vi "Configuration Tool Main.vi"() -> ()   [LabVIEW 2022 SP3, in "Configuration Tool.lvlib"]
doc: "This is the main VI for the configuration editor.Copyright 2017 National Instruments Corporation\n\nLicensed under the Apache License, Version 2.0 (the \"License\"); you may not use this file except in compliance with the License. You may obtain a copy of the License at http://www.apache.org/licenses/LICENSE-2.0\nUnless required by applicable law or agreed to in writing, software distributed under the License is distributed on an \"AS IS\" BASIS, WITHOUT WARRANTIES OR CONDITIONS OF ANY KIND, either express or implied. See the License for the specific language governing permissions and limitations under the License."
uses:
  Configuration Tool.lvlib
  Controls/StateCluster.ctl
  <vilib>/NI/Configuration Framework/Repository/NISE_CEF_Repository.lvclass
  <vilib>/NI/Configuration Framework/Node/NodeRef.ctl
  <vilib>/NI/Configuration Framework/Node/NISE_CEF_Node.lvclass
  <vilib>/NI/Configuration Framework/Node/StandardEvents.ctl
  <vilib>/NI/Configuration Framework/Node/UserEventRef.ctl
  <vilib>/NI/Configuration Framework/Controls/EventCluster.ctl
  <vilib>/NI/Configuration Framework/Node/NodeChangeEvent.ctl
  <vilib>/NI/Configuration Framework/Node/CacheState.ctl
  <vilib>/NI/Configuration Framework/Node/RefreshUIEvent.ctl
  <vilib>/NI/Configuration Framework/Node/StopEvent.ctl
  <vilib>/NI/Configuration Framework/glyph manager/glyph manager.ctl
  <vilib>/picture/picture.llb/imagedata.ctl
  Controls/AddMessage.ctl
  Controls/MoveMessage.ctl
  <vilib>/Utility/error.llb/DialogType.ctl
  Classes/cRIO Repo/BaseRepo.lvclass
  C:/Program Files (x86)/National Instruments/LabVIEW 2022/vi.lib/NI/Configuration Framework/Repository/NISE_CEF_Repository.lvclass
  Classes/BaseClass_class/BaseClass.lvclass
  <vilib>/Utility/sysdir.llb/System Directory Type.ctl
  <vilib>/NI/AMC/Create Single Message.vi
  <vilib>/NI/AMC/Update Message Routing Info.vi
  <vilib>/NI/AMC/Read Termination Message.vi
  <vilib>/NI/AMC/Send Message.vi
  <vilib>/NI/AMC/Globals.vi
  <vilib>/NI/AMC/AMC.lvlib
  <vilib>/NI/Configuration Framework/NISE_CEF_TreeControl.lvlib
  <vilib>/NI/Configuration Framework/glyph manager/glyph manager.lvlib
panel:
  in  "View":string(tree)
  in  "Exit":bool
  # "Configurator"
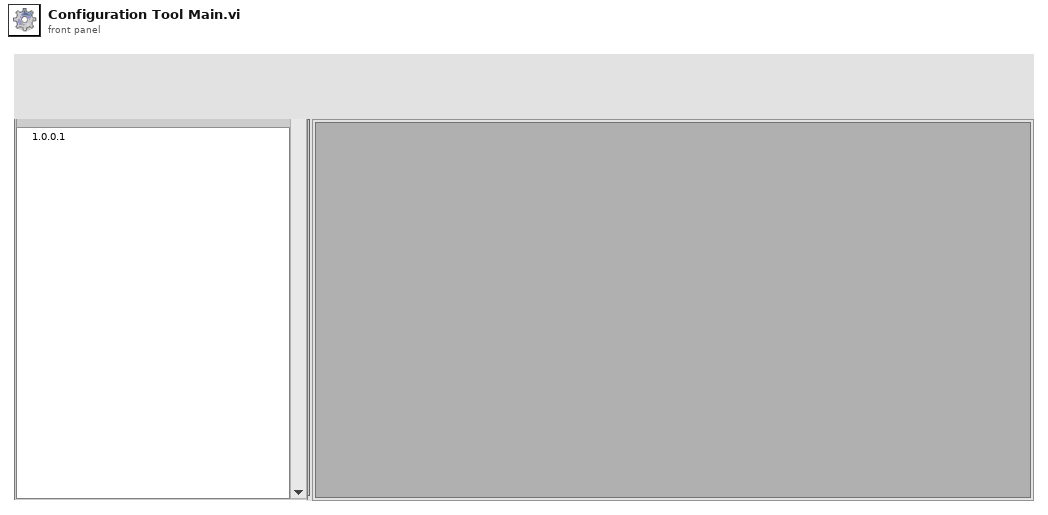
[diagram p1: front panel]
types:
  T1 = typedef "Configuration Tool.lvlib/StateCluster.ctl" = cluster{"repository":refnum<class "NISE_CEF_Repository.lvclass">, "root":T2, "unsaved changes":bool, "current path":path, "standard events":T3, "classes path":path, "glyph manager":T9}
  T2 = typedef "NISE_CEF_Node.lvclass/NodeRef.ctl" = refnum<data-value>
  T3 = typedef "NISE_CEF_Node.lvclass/StandardEvents.ctl" = cluster{"user event":T4, "node change":T5, "cache state":T6, "refresh UI":T7, "stop event":T8}
  T4 = typedef "NISE_CEF_Node.lvclass/UserEventRef.ctl" = refnum<user-event>
  T5 = typedef "NISE_CEF_Node.lvclass/NodeChangeEvent.ctl" = refnum<user-event>
  T6 = typedef "NISE_CEF_Node.lvclass/CacheState.ctl" = refnum<user-event>
  T7 = typedef "NISE_CEF_Node.lvclass/RefreshUIEvent.ctl" = refnum<user-event>
  T8 = typedef "NISE_CEF_Node.lvclass/StopEvent.ctl" = refnum<user-event>
  T9 = typedef "glyph manager.lvlib/glyph manager.ctl" = cluster{"search paths":path[], "glyph map":variant, "base glyphs":T10[], "desired overlays":string[]}
  T10 = typedef "imagedata.ctl" = cluster{"image type":i32, "image depth":i32, "image":u8[], "mask":u8[], "colors":u32[], "Rectangle":cluster{"left":i16, "top":i16, "right":i16, "bottom":i16}}
  T11 = typedef "AMC.lvlib/Message Queue.ctl" = refnum<queue>
  T12 = typedef "Configuration Tool.lvlib/AddMessage.ctl" = cluster{"node type":string, "to add to":string}
  T13 = typedef "Configuration Tool.lvlib/MoveMessage.ctl" = cluster{"node ref":T2, "new parent":T2, "Index":i32}
  T14 = typedef "Configuration Tool.lvlib/FilePaths.ctl" = cluster{"glyphs":path, "classes":path}
  T15 = typedef "DialogType.ctl" = u16
  T16 = typedef "System Directory Type.ctl" = i32
  T17 = typedef "NISE_CEF_Node.lvclass/Summary.ctl" = cluster{"ID":string, "parent ID":string, "node type":string, "text":string, "additional text":string, "glyph":string, "depth":i32, "glyph overlay":string}
  T18 = typedef "LVPoint32TypeDef.ctl" = cluster{"Horizontal":i32, "Vertical":i32}
  T19 = cluster{"data name":string, "drag data":variant}[]
  T20 = typedef "NISE_CEF_Node.lvclass/NodeMenuOptions.ctl" = cluster{"removable":bool, "movable":bool, "duplicate":bool}
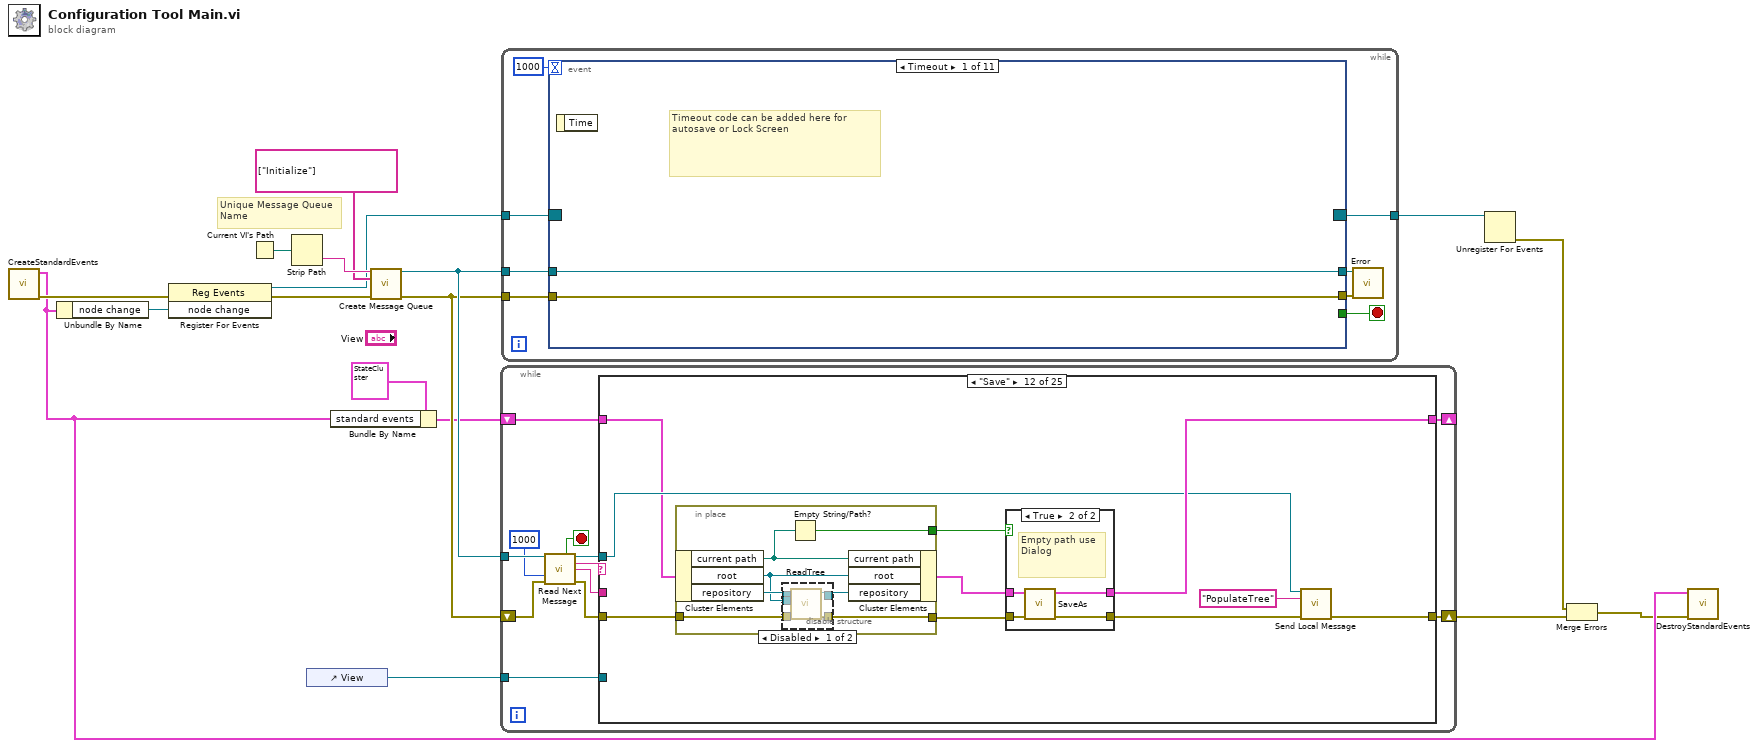
[diagram p0: block diagram]
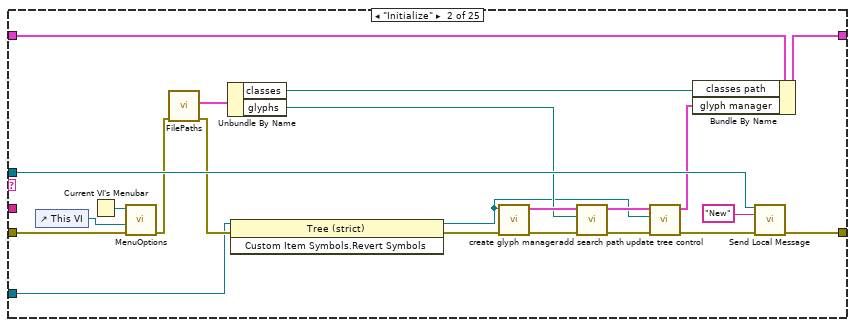
[diagram p3: hidden frame]
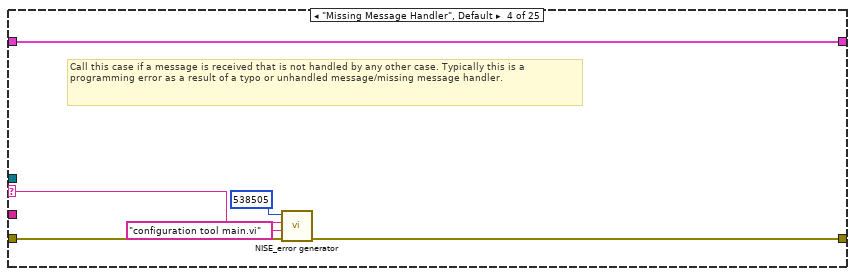
[diagram p5: hidden frame]
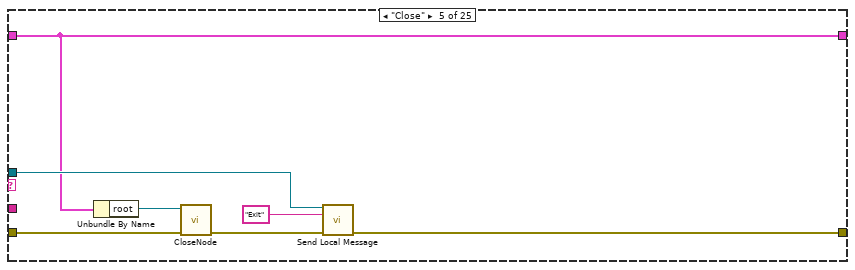
[diagram p6: hidden frame]
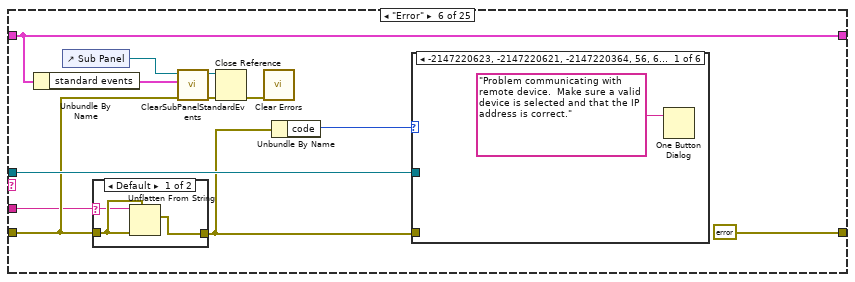
[diagram p7: hidden frame]
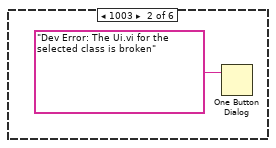
[diagram p9: hidden frame]
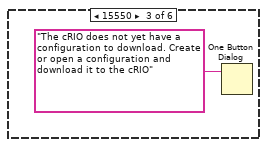
[diagram p10: hidden frame]
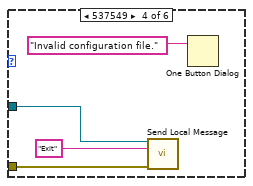
[diagram p11: hidden frame]
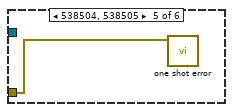
[diagram p12: hidden frame]
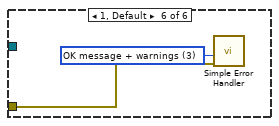
[diagram p13: hidden frame]
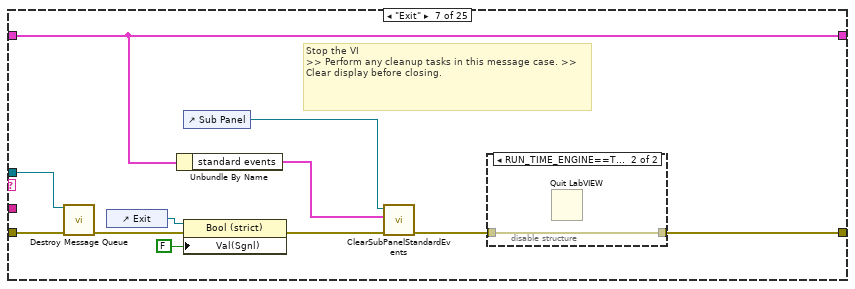
[diagram p14: hidden frame]
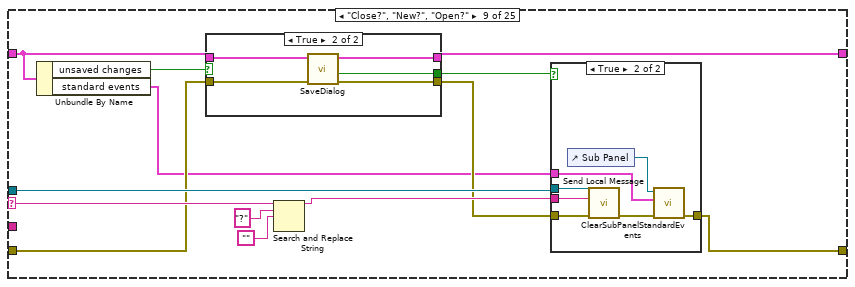
[diagram p17: hidden frame]
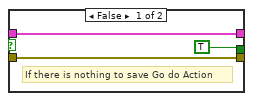
[diagram p18: hidden frame]
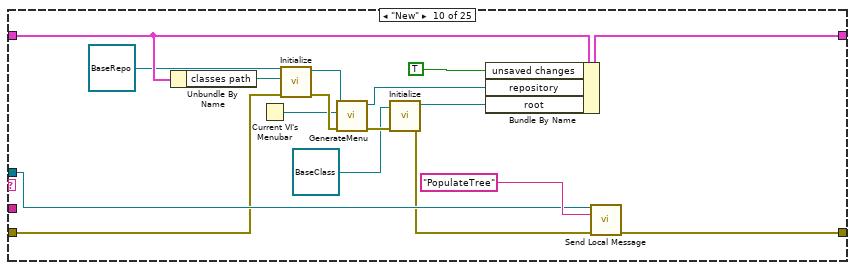
[diagram p20: hidden frame]
diagram:
  # "Unique Message Queue Name"
  n1 = call <vilib>:"CreateStandardEvents.vi"() -> ("error out"=w12:errorcluster, "standard events"=w6:T3)  [unwired: 10 in]
  n2 = Unbundle By Name(w6) -> ("node change"=w11:T5)
  n3 = register-events(error in=w12, w11) -> (reference out=w5:refnum<event-registration>, error out=w10:errorcluster)  [unwired: 1 in]
  n4 = Current VI's Path() -> (path=w16:path)
  n5 = Strip Path(path=w16) -> (name=w17:string)  [unwired: 1 out]
  n6 = control-ref of="View"() -> (w4:refnum<vi>)
  n7 = Bundle By Name(cluster=T1 {"repository"=refnum, "root"=refnum, "unsaved changes"=FALSE, "current path"=path "", "standard events"={"user event"=refnum, "node change"=refnum, "cache state"=refnum, "refresh UI"=refnum, "stop event"=refnum}, "classes path"=path "", "glyph manager"={"search paths"=[], "glyph map"=variant, "base glyphs"=[], "desired overlays"=[]}}, "standard events"=w6) -> (w8:T1)
  n8 = call <vilib>:"Create Message Queue.vi"("message queue name"=w17, "initial message names"=string[] ["Initialize"], "error in"=w10) -> ("message queue out"=w14:T11, "error out"=w13:errorcluster)  [unwired: 11 in]
  n9 = while "Message Processor" {
    shift-right: [w25] -> w7
    shift-left: w13 -> [w24]
    tunnel: w14 -> [w23]
    shift-right: [w21] -> _
    shift-left: w8 -> [w20]
    tunnel: w4 -> [w18]
    stop <- w29 stop-if-true
    n10 = call <vilib>:"Read Next Message.vi"("message queue in"=w23, "timeout (1 ms)"=1000, "error in"=w24) -> ("exit process?"=w29:bool, "message queue out"=w19:T11, "message name"=w28:string, "message value"=w27:string, "error out"=w26:errorcluster)  [unwired: 5 in, 3 out]
    n11 = case shown="\"Save\"" w28 {
      selector: w28 -> [_ _ _ w57 _ _ _ _ w118 _ _ _ _ _ _ _ _ w335 _ _ _ _ _ _ _]
      tunnel: w27 -> [_ _ _ _ _ w70 _ _ _ _ _ _ _ w246 _ w296 w313 w333 w385 w409 _ _ w449 w470 w477]
      tunnel: w26 -> [w31 w53 w55 w60 w63 w73 w105 w109 w111 w146 w162 w202 w233 w253 w273 w288 w312 w338 w387 w408 w430 w439 w448 w468 w478]
      tunnel: [w31 w49 w55 w58 w67 errorcluster {"status"=FALSE, "code"=0, "source"=""} ("error out") w97 w109 w122 w154 w158 w206 w235 w250 w273 w290 w316 w341 w389 w405 w424 w435 w445 w463 w476] -> w25
      tunnel: [w30 w45 w54 w61 w65 w77 w96 w108 w113 w152 w163 w209 w234 w247 w272 w282 w309 w342 w388 w410 w421 w438 w443 w471 w473] -> w21
      tunnel: w20 -> [w30 w46 w54 w61 w65 w77 w96 w108 w114 w149 w164 w204 w232 w248 w272 w286 w310 w342 w380 w410 w433 w438 w443 w471 w479]
      tunnel: w19 -> [_ w48 _ _ w66 w80 w104 _ w121 w153 w160 w205 _ w249 _ _ _ w336 _ _ _ _ w444 w462 w475]
      tunnel: w18 -> [_ w32 _ _ _ _ _ _ _ _ _ _ _ _ _ w283 w305 w330 w382 w403 w422 _ _ _ _]
      frame "------------Generic Operations------------" {
        # "Dummy case to add a seperation in the Case Structure menu"
      }
      frame "Initialize" {
        n12 = control-ref of="This VI"() -> (w52:refnum<vi>)
        n13 = Current VI's Menubar() -> (w51:refnum<k9>)
        n14 = call "MenuOptions.vi"("error in"=w53, "VI ref"=w52, "menu ref in"=w51) -> ("error out"=w44:errorcluster)  [unwired: 7 in, 1 out]
        n15 = call "FilePaths.vi"("error in"=w44) -> ("error out"=w35:errorcluster, "paths"=w47:T14)  [unwired: 9 in]
        n16 = Unbundle By Name(w47) -> ("classes"=w43:path, "glyphs"=w37:path)
        n17 = invoke class="Tree (strict)" method="Custom Item Symbols.Revert Symbols"(reference=w32, error in=w35) -> (reference out=w33:refnum<vi>, error out=w34:errorcluster)  [unwired: 1 in, 1 out]
        n18 = call <vilib>:"create glyph manager.vi"("error in"=w34, "tree ref (for default symbols)"=w33) -> ("error out"=w42:errorcluster, "glyph manager"=w41:T9)  [unwired: 8 in]
        n19 = call <vilib>:"add search path.vi"("error in"=w42, "search path"=w37, "glyph manager in"=w41) -> ("error out"=w40:errorcluster, "glyph manager out"=w39:T9)  [unwired: 7 in]
        n20 = call <vilib>:"update tree control.vi"("error in"=w40, "tree reference"=w33, "glyph manager in"=w39) -> ("error out"=w38:errorcluster, "glyph manager out"=w36:T9)  [unwired: 7 in]
        n21 = Bundle By Name(cluster=w46, "classes path"=w43, "glyph manager"=w36) -> (w45:T1)
        n22 = call <vilib>:"Send Local Message.vi"("message queue in"=w48, "message name"="New" ("Message Name"), "error in"=w38) -> ("error out"=w49:errorcluster)  [unwired: 10 in, 2 out]
      }
      frame "", "Idle" {
      }
      frame "Missing Message Handler", Default {
        # "Call this case if a message is received that is not handled by any other case. Typically this is a programming error as a result of a typo or unhandled message/missing message handler."
        n23 = call <vilib>:"NISE_error generator.vi"("error in"=w60, "source"="configuration tool main.vi", "append error message"=w57, "error code (0)"=538505) -> ("error out"=w58:errorcluster)  [unwired: 5 in]
      }
      frame "Close" {
        n24 = Unbundle By Name(w65) -> ("root"=w64:T2)
        n25 = call <vilib>:"CloseNode.vi"("error in"=w63, "node ref"=w64) -> ("error out"=w62:errorcluster)  [unwired: 9 in]
        n26 = call <vilib>:"Send Local Message.vi"("message queue in"=w66, "message name"="Exit", "error in"=w62) -> ("error out"=w67:errorcluster)  [unwired: 10 in, 2 out]
      }
      frame "Error" {
        n27 = Unbundle By Name(w77) -> ("standard events"=w69:T3)
        n28 = control-ref of="Sub Panel"() -> (w76:refnum<vi>)
        n29 = case shown="Default" w70 {
          selector: w70 -> [w82 _]
          tunnel: w73 -> [w83 w84]
          tunnel: [w81 w84] -> w72
          frame Default {
            n30 = Unflatten From String(type=w83, binary string=w82, error in (no error)=w83) -> (value=w81:errorcluster)  [unwired: 2 in, 2 out]
          }
          frame "" {
          }
        }
        n31 = call <vilib>:"ClearSubPanelStandardEvents.vi"("error in"=w73, "standard events"=w69, "sub panel ref in"=w76) -> ("error out"=w75:errorcluster, "sub panel ref out"=w74:refnum<vi>)  [unwired: 7 in]
        n32 = Close Reference(reference=w74, error in (no error)=w75) -> (error out=w71:errorcluster)
        n33 = call <vilib>:"Clear Errors.vi"("error in (no error)"=w71) -> ()  [unwired: 5 in, 2 out]
        n34 = Unbundle By Name(w72) -> ("code"=w78:i32)
        n35 = case shown="-2147220623, -2147220621, -2147220364, 56, 63" w78 {
          tunnel: w80 -> [_ _ _ w90 _ _]
          tunnel: w72 -> [_ _ _ w89 w92 w94]
          frame -2147220623, -2147220621, -2147220364, 56, 63 {
            n36 = One Button Dialog(message="Problem communicating with remote device.  Make sure a valid device is selected and that the IP address is correct.") -> ()  [unwired: 1 in, 1 out]
          }
          frame 1003 {
            n37 = One Button Dialog(message="Dev Error: The Ui.vi for the selected class is broken") -> ()  [unwired: 1 in, 1 out]
          }
          frame 15550 {
            n38 = One Button Dialog(message="The cRIO does not yet have a configuration to download. Create or open a configuration and download it to the cRIO") -> ()  [unwired: 1 in, 1 out]
          }
          frame 537549 {
            n39 = call <vilib>:"Send Local Message.vi"("message queue in"=w90, "message name"="Exit", "error in"=w89) -> ()  [unwired: 10 in, 3 out]
            n40 = One Button Dialog(message="Invalid configuration file.") -> ()  [unwired: 1 in, 1 out]
          }
          frame 538504, 538505 {
            n41 = call <vilib>:"one shot error.vi"("error in"=w92) -> ()  [unwired: 11 in]
          }
          frame 1, Default {
            w93 = T15 3 items=["no dialog", "OK message", "continue or stop message", "OK message + warnings", "continue/stop + warnings"] ("type of dialog (OK msg:1)")
            n42 = call <vilib>:"Simple Error Handler.vi"("type of dialog (OK msg:1)"=w93, "error in (no error)"=w94) -> ()  [unwired: 8 out]
          }
        }
      }
      frame "Exit" {
        # "Stop the VI                                                                             >> Perform any cleanup tasks in this message case. >> Clear display before closing."
        n43 = call <vilib>:"Destroy Message Queue.vi"("message queue in"=w104, "error in"=w105) -> ("error out"=w101:errorcluster)  [unwired: 11 in, 2 out]
        n44 = control-ref of="Exit"() -> (w103:refnum<vi>)
        n45 = Unbundle By Name(w96) -> ("standard events"=w95:T3)
        n46 = control-ref of="Sub Panel"() -> (w100:refnum<vi>)
        n47 = property class="Bool (strict)"(reference=w103, error in=w101, "Val(Sgnl)"=FALSE ("Exit")) -> (error out=w99:errorcluster)  [unwired: 1 out]
        n48 = call <vilib>:"ClearSubPanelStandardEvents.vi"("error in"=w99, "standard events"=w95, "sub panel ref in"=w100) -> ("error out"=w98:errorcluster)  [unwired: 7 in, 1 out]
        n49 = disable-structure shown="RUN_TIME_ENGINE==True" {
          disable-tunnel: [w106 w107] -> w97
          disable-tunnel: w98 -> [w106 w107]
          frame condition #0 (active) {
          }
          frame condition #1 {
            n50 = Quit LabVIEW() -> ()  [unwired: 1 in]
          }
        }
      }
      frame "------------Menu Operations--------------" {
        # "Dummy case to add a seperation in the Case Structure menu"
      }
      frame "Close?", "New?", "Open?" {
        n51 = Unbundle By Name(w114) -> ("unsaved changes"=w116:bool, "standard events"=w110:T3)
        n52 = case shown="True" w116 {
          tunnel: [TRUE ("SaveFlag") w130] -> w115
          tunnel: w114 -> [w124 w129]
          tunnel: [w124 w128] -> w113
          tunnel: w111 -> [w123 w127]
          tunnel: [w123 w126] -> w112
          frame False {
            # "If there is nothing to save Go do Action"
          }
          frame True {
            n53 = call "SaveDialog.vi"("error in"=w127, "state in"=w129) -> ("error out"=w126:errorcluster, "new"=w130:bool, "state out"=w128:T1)  [unwired: 7 in]
          }
        }
        n54 = Search and Replace String(input string=w118, search string="?", replace string="") -> (result string=w117:string)  [unwired: 5 in, 3 out]
        n55 = case shown="True" w115 {
          tunnel: w112 -> [w131 w138]
          tunnel: [w131 w134] -> w122
          tunnel: w121 -> [_ w137]
          tunnel: w117 -> [_ w136]
          tunnel: w110 -> [_ w132]
          frame False {
          }
          frame True {
            n56 = control-ref of="Sub Panel"() -> (w133:refnum<vi>)
            n57 = call <vilib>:"Send Local Message.vi"("message queue in"=w137, "message name"=w136, "error in"=w138) -> ("error out"=w135:errorcluster)  [unwired: 10 in, 2 out]
            n58 = call <vilib>:"ClearSubPanelStandardEvents.vi"("error in"=w135, "standard events"=w132, "sub panel ref in"=w133) -> ("error out"=w134:errorcluster)  [unwired: 7 in, 1 out]
          }
        }
      }
      frame "New" {
        n59 = Unbundle By Name(w149) -> ("classes path"=w148:path)
        n60 = Current VI's Menubar() -> (w141:refnum<k9>)
        n61 = call-dynamic "Initialize.vi"("error in"=w146, "path"=w148, "repository in"=refnum<class "BaseRepo.lvclass"> refnum ("BaseRepo.lvclass")) -> ("error out"=w145:errorcluster, "repository out"=w143:refnum<class "BaseRepo.lvclass">)  [unwired: 7 in]
        n62 = call-dynamic "GenerateMenu.vi"("error in"=w145, "menu ref in"=w141, "NISE_CEF_Repository in"=w143) -> ("error out"=w144:errorcluster, "NISE_CEF_Repository out"=w142:refnum<class "BaseRepo.lvclass">)  [unwired: 6 in, 1 out]
        n63 = call-dynamic "Initialize.vi"("error in"=w144, "cRIO in"=refnum<class "BaseClass.lvclass"> refnum ("BaseClass.lvclass")) -> ("error out"=w147:errorcluster, "data value reference"=w150:T2)  [unwired: 7 in, 1 out]
        n64 = Bundle By Name(cluster=w149, "unsaved changes"=TRUE ("SaveFlag"), "repository"=w142, "root"=w150) -> (w152:T1)
        n65 = call <vilib>:"Send Local Message.vi"("message queue in"=w153, "message name"="PopulateTree", "error in"=w147) -> ("error out"=w154:errorcluster)  [unwired: 10 in, 2 out]
      }
      frame "Open" {
        w157 = T16 0 items=["User Home"=0, "User Desktop"=1, "User Documents"=2, "User Application Data"=3, "User Preferences"=4, "User Temporary"=5, "Public Documents"=6, "Public Application Data"=7, "Public Preferences"=8, "Public Cache"=13, "System Core Libraries"=9, "System Installed Libraries"=10, "Application Files"=11, "Boot Volume Root"=12] ("system directory type")
        n66 = call <vilib>:"Get System Directory.vi"("system directory type"=w157) -> ("system directory"=w156:path)  [unwired: 10 in]
        n67 = in-place {
          in-place-border: w162 -> [w170]
          in-place-border: [w169] -> w159
          in-place-border: w156 -> [w165]
          n68 = in-place-cluster #1(w164) -> ("current path"=w167:path, "repository"=w178:refnum<class "NISE_CEF_Repository.lvclass">, "root"=w174:T2)  [unwired: 1 out]
          n69 = call "FileDialog.vi"("error in"=w170, "start path"=w165) -> ("error out"=w171:errorcluster, "cancelled"=w172:bool, "selected path"=w168:path)  [unwired: 7 in]
          n70 = Compound Arithmetic op=OR(invert w172) -> (w173:bool)
          n71 = case shown="True" w173 {
            tunnel: w178 -> [w179 w191]
            tunnel: [w179 w189] -> w176
            tunnel: [w180 w187] -> w169
            tunnel: [w181 w186] -> w175
            tunnel: w168 -> [_ w184]
            tunnel: w171 -> [w180 w183]
            tunnel: w174 -> [w181 w182]
            frame False {
            }
            frame True {
              n72 = call-dynamic "Open.vi"("error in"=w183, "file path"=w184, "repository in"=w191) -> ("error out"=w188:errorcluster, "invalid?"=w185:bool, "repository out"=w190:refnum<class "NISE_CEF_Repository.lvclass">)  [unwired: 6 in]
              n73 = case shown="False" w185 {
                tunnel: w190 -> [w196 w199]
                tunnel: [w195 w199] -> w189
                tunnel: w188 -> [w194 w198]
                tunnel: [w193 w198] -> w187
                tunnel: [w192 w197] -> w186
                tunnel: w182 -> [_ w197]
                frame False {
                  n74 = call-dynamic "WriteTree.vi"("error in"=w194, "repository in"=w196) -> ("error out"=w193:errorcluster, "root"=w192:T2, "repository out"=w195:refnum<class "NISE_CEF_Repository.lvclass">)  [unwired: 7 in]
                }
                frame True {
                }
              }
            }
          }
          n75 = Select(t=w167, s=w169, f=w168) -> (s? t:f=w166:path)
          n76 = in-place-cluster #1("current path"=w166, "unsaved changes"=FALSE ("SaveFlag"), "repository"=w176, "root"=w175) -> (w163:T1)
        }
        n77 = call <vilib>:"Send Local Message.vi"("message queue in"=w160, "message name"="PopulateTree", "error in"=w159) -> ("error out"=w158:errorcluster)  [unwired: 10 in, 2 out]
      }
      frame "Save" {
        n78 = in-place {
          in-place-border: w202 -> [w213]
          in-place-border: [w212] -> w201
          in-place-border: [w210] -> w200
          n79 = in-place-cluster #2(w204) -> ("current path"=w211:path, "root"=w214:T2, "repository"=w216:refnum<class "NISE_CEF_Repository.lvclass">)
          n80 = disable-structure shown="Disabled" {
            disable-tunnel: w216 -> [w221 _]
            disable-tunnel: [w220 _] -> w215
            disable-tunnel: w214 -> [w219 _]
            disable-tunnel: w213 -> [w218 _]
            disable-tunnel: [w217 _] -> w212
            frame Disabled {
              n81 = call-dynamic "ReadTree.vi"("error in"=w218, "root"=w219, "repository in"=w221) -> ("error out"=w217:errorcluster, "repository out"=w220:refnum<class "NISE_CEF_Repository.lvclass">)  [unwired: 7 in]
            }
            frame Enabled {
            }
          }
          n82 = Empty String/Path?(string/path=w211) -> (empty?=w210:bool)
          n83 = in-place-cluster #2("current path"=w211, "root"=w214, "repository"=w215) -> (w203:T1)
        }
        n84 = case shown="True" w200 {
          tunnel: w203 -> [w225 w227]
          tunnel: [w224 w226] -> w209
          tunnel: [w223 w228] -> w207
          tunnel: w201 -> [w222 w229]
          frame False {
            n85 = call "Save.vi"("error in"=w222, "state in"=w225) -> ("error out"=w223:errorcluster, "state out"=w224:T1)  [unwired: 8 in]
          }
          frame True {
            # "Empty path use Dialog"
            n86 = call "SaveAs.vi"("error in"=w229, "state in"=w227) -> ("error out"=w228:errorcluster, "state out"=w226:T1)  [unwired: 7 in, 1 out]
          }
        }
        n87 = call <vilib>:"Send Local Message.vi"("message queue in"=w205, "message name"="PopulateTree", "error in"=w207) -> ("error out"=w206:errorcluster)  [unwired: 10 in, 2 out]
      }
      frame "SaveAs" {
        n88 = in-place {
          in-place-border: w233 -> [w237]
          in-place-border: [w236] -> w231
          n89 = in-place-cluster #3(w232) -> ("root"=w238:T2, "repository"=w240:refnum<class "NISE_CEF_Repository.lvclass">)
          n90 = disable-structure shown="Disabled" {
            disable-tunnel: w240 -> [w245 _]
            disable-tunnel: [w244 _] -> w239
            disable-tunnel: w238 -> [w243 _]
            disable-tunnel: w237 -> [w242 _]
            disable-tunnel: [w241 _] -> w236
            frame Disabled {
              n91 = call-dynamic "ReadTree.vi"("error in"=w242, "root"=w243, "repository in"=w245) -> ("error out"=w241:errorcluster, "repository out"=w244:refnum<class "NISE_CEF_Repository.lvclass">)  [unwired: 7 in]
            }
            frame Enabled {
            }
          }
          n92 = in-place-cluster #3("root"=w238, "repository"=w239) -> (w230:T1)
        }
        n93 = call "SaveAs.vi"("error in"=w231, "state in"=w230) -> ("error out"=w235:errorcluster, "state out"=w234:T1)  [unwired: 7 in, 1 out]
      }
      frame "Custom View" {
        n94 = in-place {
          in-place-border: w253 -> [w260]
          in-place-border: [w259] -> w251
          in-place-border: w246 -> [w254]
          n95 = in-place-cluster #4(w248) -> ("repository"=w258:refnum<class "NISE_CEF_Repository.lvclass">, "root"=w257:T2)
          n96 = disable-structure shown="Disabled" {
            disable-tunnel: w260 -> [w271 _]
            disable-tunnel: [w270 _] -> w259
            disable-tunnel: w258 -> [w265 _]
            disable-tunnel: w257 -> [w264 _]
            disable-tunnel: [w263 _] -> w256
            disable-tunnel: [w262 _] -> w255
            disable-tunnel: w254 -> [w261 _]
            frame Disabled {
              n97 = call-dynamic "ReadTree.vi"("error in"=w271, "root"=w264, "repository in"=w265) -> ("error out"=w268:errorcluster, "repository out"=w267:refnum<class "NISE_CEF_Repository.lvclass">)  [unwired: 7 in]
              n98 = call-dynamic "CustomView.vi"("error in"=w268, "view name"=w261, "repository in"=w267) -> ("error out"=w269:errorcluster, "repository out"=w266:refnum<class "NISE_CEF_Repository.lvclass">)  [unwired: 7 in]
              n99 = call-dynamic "WriteTree.vi"("error in"=w269, "repository in"=w266) -> ("error out"=w270:errorcluster, "root"=w262:T2, "repository out"=w263:refnum<class "NISE_CEF_Repository.lvclass">)  [unwired: 7 in]
            }
            frame Enabled {
            }
          }
          n100 = in-place-cluster #4("repository"=w256, "root"=w255) -> (w247:T1)
        }
        n101 = call <vilib>:"Send Local Message.vi"("message queue in"=w249, "message name"="PopulateTree", "error in"=w251) -> ("error out"=w250:errorcluster)  [unwired: 10 in, 2 out]
      }
      frame "-------TreeControl Operations-----------" {
        # "Dummy case to add a seperation in the Case Structure menu"
      }
      frame "AddNode" {
        n102 = Unflatten From String(type=T12 {"node type"="", "to add to"=""} ("input cluster"), binary string=w296) -> (value=w294:T12)  [unwired: 3 in, 2 out]
        n103 = Unbundle By Name(w294) -> ("to add to"=w292:string, "node type"=w285:string)
        n104 = in-place {
          in-place-border: w288 -> [w302]
          in-place-border: [w301] -> w287
          in-place-border: w285 -> [w300]
          in-place-border: [w299] -> w284
          n105 = in-place-cluster #5(w286) -> ("repository"=w304:refnum<class "NISE_CEF_Repository.lvclass">)
          n106 = call-dynamic "GetClassPath.vi"("error in"=w302, "class name"=w300, "Repository in"=w304) -> ("error out"=w301:errorcluster, "class path"=w299:path, "Repository out"=w303:refnum<class "NISE_CEF_Repository.lvclass">)  [unwired: 6 in]
          n107 = in-place-cluster #5("repository"=w303) -> (w279:T1)
        }
        n108 = Unbundle By Name(w279) -> ("glyph manager"=w278:T9)
        n109 = call <vilib>:"Get LV Class Default Value.vi"("error in (no error)"=w287, "class path"=w284) -> ("error out"=w297:errorcluster, "object"=w298:refnum<class>)  [unwired: 8 in]
        n110 = To More Specific Class(target class=refnum<class "NISE_CEF_Node.lvclass"> refnum ("Node.lvclass"), reference=w298, error in=w297) -> (specific class reference=w280:refnum<class "NISE_CEF_Node.lvclass">, error out=w281:errorcluster)
        n111 = call-dynamic "AddGlyphtoGManager.vi"("error in"=w281, "glyph manager"=w278, "NISE_CEF_Node in"=w280) -> ("error out"=w276:errorcluster, "glyph manager out"=w277:T9, "NISE_CEF_Node out"=w275:refnum<class "NISE_CEF_Node.lvclass">)  [unwired: 6 in]
        n112 = call <vilib>:"AddNode.vi"("error in"=w276, "node in"=w275, "parent node ID"=w292) -> ("error out"=w291:errorcluster, "summary"=w289:T17[])  [unwired: 7 in]
        n113 = call <vilib>:"PopulateTreeSumaryWithGlyphManager.vi"("error in"=w291, "glyph manager"=w277, "summary"=w289, "tree ref in"=w283) -> ("error out"=w290:errorcluster, "glyph manager out"=w274:T9)  [unwired: 6 in]
        n114 = Bundle By Name(cluster=w279, "glyph manager"=w274) -> (w282:T1)
      }
      frame "Duplicate" {
        n115 = call <vilib>:"IDtoNode.vi"("error in"=w312, "ID"=w313) -> ("error out"=w314:errorcluster, "invalid Id"=w311:bool, "node ref"=w315:T2)  [unwired: 7 in]
        n116 = Unbundle By Name(w310) -> ("glyph manager"=w307:T9)
        n117 = case shown="False" w311 {
          tunnel: [w327 w329] -> w316
          tunnel: w315 -> [w326 _]
          tunnel: w314 -> [w323 w329]
          tunnel: w307 -> [w319 w328]
          tunnel: [w318 w328] -> w306
          tunnel: w305 -> [w317 _]
          frame False {
            n118 = call <vilib>:"DuplicateNode.vi"("same parent?"=TRUE ("s"), "error in"=w323, "node ref in"=w326) -> ("error out"=w324:errorcluster, "new node ref"=w325:T2)  [unwired: 7 in]
            n119 = call <vilib>:"Summary.vi"("error in"=w324, "node self ref"=w325) -> ("error out"=w321:errorcluster, "summary"=w320:T17[])  [unwired: 8 in]
            n120 = call <vilib>:"PopulateTreeSumaryWithGlyphManager.vi"("error in"=w321, "glyph manager"=w319, "summary"=w320, "tree ref in"=w317) -> ("error out"=w327:errorcluster, "glyph manager out"=w318:T9)  [unwired: 6 in]
          }
          frame True {
          }
        }
        n121 = Bundle By Name(cluster=w310, "unsaved changes"=TRUE, "glyph manager"=w306) -> (w309:T1)
      }
      frame "CustomMenuAction" {
        n122 = Match Pattern(string=w333, regular expression=":") -> (before substring=w332:string, after substring=w331:string)  [unwired: 1 in, 2 out]
        n123 = call <vilib>:"IDtoNode.vi"("error in"=w338, "ID"=w331) -> ("error out"=w339:errorcluster, "invalid Id"=w337:bool, "node ref"=w340:T2)  [unwired: 7 in]
        n124 = case shown="False" w337 {
          tunnel: [w348 w378] -> w341
          tunnel: w340 -> [w345 _]
          tunnel: w339 -> [w351 w378]
          tunnel: w336 -> [w352 _]
          tunnel: w335 -> [_ _]
          tunnel: w332 -> [w349 _]
          tunnel: w330 -> [w346 _]
          frame False {
            n125 = in-place {
              in-place-border: w352 -> [w376]
              in-place-border: w351 -> [w374]
              in-place-border: [w373] -> w347
              in-place-border: [w372] -> w350
              in-place-border: w349 -> [w371]
              in-place-border: w346 -> [w370]
              in-place-border: [w369] -> w344
              n126 = in-place-dvr #6(w345) -> (w377:refnum<class "NISE_CEF_Node.lvclass">)  [unwired: 1 out]
              n127 = call-dynamic "MenuHandler.vi"("tree control"=w370, "main message queue"=w376, "error in"=w374, "menu string"=w371, "NISE_CEF_Node in"=w377) -> ("error out"=w373:errorcluster, "refresh tree?"=w369:bool, "Unhandled"=w372:bool, "NISE_CEF_Node out"=w375:refnum<class "NISE_CEF_Node.lvclass">)  [unwired: 3 in]
              n128 = in-place-dvr #6(w375) -> (w343:T2)  [unwired: 1 out]
            }
            n129 = case shown="False" w350 {
              tunnel: w349 -> [_ w364]
              tunnel: [w356 w365] -> w348
              tunnel: w347 -> [w354 w366]
              tunnel: w344 -> [w353 _]
              tunnel: w343 -> [w355 _]
              frame False {
                n130 = case shown="True" w353 {
                  tunnel: [w357 w360] -> w356
                  tunnel: w355 -> [_ w359]
                  tunnel: w354 -> [w357 w358]
                  frame False {
                  }
                  frame True {
                    n131 = call <vilib>:"NodetoID.vi"("error in"=w358, "node ref"=w359) -> ("error out"=w362:errorcluster, "ID"=w363:string)  [unwired: 8 in]
                    n132 = call <vilib>:"Send Local Message.vi"("message name"="NodeDataChange", "message value"=w363, "error in"=w362) -> ("error out"=w360:errorcluster)  [unwired: 10 in, 2 out]
                  }
                }
              }
              frame True {
                n133 = call <vilib>:"NISE_error generator.vi"("error in"=w366, "source"="configuration tool main.vi", "append error message"=w364, "error code (0)"=538506) -> ("error out"=w365:errorcluster)  [unwired: 5 in]
              }
            }
          }
          frame True {
          }
        }
      }
      frame "RefreshNode" {
        # "Refreshes the node in the Tree, Sets the save flag to true. This case can be called from the UIs of the nodes"
        n134 = Unbundle By Name(w380) -> ("glyph manager"=w379:T9)
        n135 = call <vilib>:"IDtoNode.vi"("error in"=w387, "ID"=w385) -> ("error out"=w386:errorcluster, "invalid Id"=w383:bool, "node ref"=w384:T2)  [unwired: 7 in]
        n136 = case shown="False" w383 {
          tunnel: [w399 w402] -> w389
          tunnel: w386 -> [w395 w402]
          tunnel: w384 -> [w394 _]
          tunnel: w382 -> [w393 _]
          tunnel: [w392 w401] -> w381
          tunnel: w379 -> [w390 w401]
          frame False {
            n137 = call <vilib>:"SummaryWithGlyphManager.vi"("error in"=w395, "glyph manager"=w390, "node self ref"=w394) -> ("error out"=w397:errorcluster, "glyph manager out"=w391:T9, "summary"=w396:T17[])  [unwired: 6 in]
            n138 = call <vilib>:"RefreshSubTreeWithGlyphManager.vi"("error in"=w397, "glyph manager"=w391, "node information"=w396, "tree ref in"=w393) -> ("error out"=w400:errorcluster, "glyph manager out"=w392:T9, "tree ref out"=w398:refnum<vi>)  [unwired: 5 in]
            n139 = Close Reference(reference=w398, error in (no error)=w400) -> (error out=w399:errorcluster)
          }
          frame True {
          }
        }
        n140 = Bundle By Name(cluster=w380, "glyph manager"=w381) -> (w388:T1)
      }
      frame "RemoveNode" {
        n141 = call <vilib>:"IDtoNode.vi"("error in"=w408, "ID"=w409) -> ("error out"=w407:errorcluster, "invalid Id"=w404:bool, "node ref"=w406:T2)  [unwired: 7 in]
        n142 = case shown="False" w404 {
          tunnel: w407 -> [w416 w417]
          tunnel: w406 -> [w415 _]
          tunnel: [w412 w417] -> w405
          tunnel: w403 -> [w411 _]
          frame False {
            n143 = call <vilib>:"RemoveNode.vi"("error in"=w416, "node"=w415) -> ("error out"=w413:errorcluster, "node ID"=w414:string)  [unwired: 8 in]
            n144 = call <vilib>:"ClearTreeNode.vi"("error in"=w413, "tag"=w414, "tree reference"=w411) -> ("error out"=w412:errorcluster)  [unwired: 8 in]
          }
          frame True {
          }
        }
      }
      frame "PopulateTree" {
        n145 = Unbundle By Name(w433) -> ("standard events"=w423:T3, "glyph manager"=w419:T9, "root"=w428:T2)
        n146 = call <vilib>:"SummaryWithGlyphManager.vi"("error in"=w430, "glyph manager"=w419, "depth"=0 ("Depth"), "node self ref"=w428) -> ("error out"=w429:errorcluster, "glyph manager out"=w418:T9, "summary"=w432:T17[])  [unwired: 5 in]
        n147 = control-ref of="This VI"() -> (w431:refnum<vi>)
        n148 = call <vilib>:"RefreshEntireTreeWithGlyphManager.vi"("calling VI in"=w431, "error in"=w429, "glyph manager"=w418, "array"=w432, "tree ref in"=w422) -> ("error out"=w425:errorcluster, "glyph manager out"=w420:T9)  [unwired: 5 in]
        n149 = control-ref of="Sub Panel"() -> (w426:refnum<vi>)
        n150 = Bundle By Name(cluster=w433, "glyph manager"=w420) -> (w421:T1)
        n151 = call <vilib>:"ClearSubPanelStandardEvents.vi"("error in"=w425, "standard events"=w423, "sub panel ref in"=w426) -> ("error out"=w424:errorcluster)  [unwired: 7 in, 1 out]
      }
      frame "CleansubPanel" {
        n152 = Unbundle By Name(w438) -> ("standard events"=w434:T3)
        n153 = control-ref of="Sub Panel"() -> (w440:refnum<vi>)
        n154 = call <vilib>:"ClearSubPanelStandardEvents.vi"("error in"=w439, "standard events"=w434, "sub panel ref in"=w440) -> ("error out"=w437:errorcluster, "sub panel ref out"=w436:refnum<vi>)  [unwired: 7 in]
        n155 = Close Reference(reference=w436, error in (no error)=w437) -> (error out=w435:errorcluster)
      }
      frame "ActivateNode" {
        n156 = Unbundle By Name(w443) -> ("standard events"=w442:T3)
        n157 = call <vilib>:"IDtoNode.vi"("error in"=w448, "ID"=w449) -> ("error out"=w441:errorcluster, "invalid Id"=w447:bool, "node ref"=w446:T2)  [unwired: 7 in]
        n158 = case shown="False" w447 {
          tunnel: w446 -> [w456 _]
          tunnel: [w457 w458] -> w445
          tunnel: w441 -> [w454 w458]
          tunnel: w444 -> [w452 _]
          tunnel: w442 -> [w450 _]
          frame False {
            n159 = control-ref of="Sub Panel"() -> (w453:refnum<vi>)
            n160 = call <vilib>:"ClearSubPanelStandardEvents.vi"("error in"=w454, "standard events"=w450, "sub panel ref in"=w453) -> ("error out"=w455:errorcluster, "sub panel ref out"=w451:refnum<vi>)  [unwired: 7 in]
            n161 = call <vilib>:"LoadNodeUIStandardEvents.vi"("user event out"=w450, "error in"=w455, "sub panel ref in"=w451, "main queue"=w452, "node"=w456) -> ("error out"=w457:errorcluster)  [unwired: 6 in]
          }
          frame True {
          }
        }
      }
      frame "Move" {
        n162 = Unflatten From String(type=T13 {"node ref"=refnum, "new parent"=refnum, "Index"=0} ("Cluster"), binary string=w470, error in (no error)=w468) -> (value=w467:T13, error out=w466:errorcluster)  [unwired: 2 in, 1 out]
        n163 = Unbundle By Name(w467) -> ("node ref"=w461:T2, "new parent"=w460:T2, "Index"=w459:i32)
        n164 = call <vilib>:"MoveNode.vi"("error in"=w466, "index"=w459, "new parent"=w460, "node"=w461) -> ("error out"=w464:errorcluster)  [unwired: 7 in]
        n165 = call <vilib>:"Send Local Message.vi"("message queue in"=w462, "message name"="PopulateTree", "error in"=w464) -> ("error out"=w463:errorcluster)  [unwired: 10 in, 2 out]
      }
      frame "NodeDataChange" {
        n166 = call <vilib>:"Send Local Message.vi"("message queue in"=w475, "message name"="RefreshNode", "message value"=w477, "error in"=w478) -> ("error out"=w476:errorcluster)  [unwired: 9 in, 2 out]
        n167 = Bundle By Name(cluster=w479, "unsaved changes"=TRUE) -> (w473:T1)
      }
    }
  }
  n168 = while "User Interface Event Handler" {
    tunnel: w14 -> [w486]
    tunnel: w13 -> [w482]
    tunnel: w5 -> [w481]
    tunnel: [w480] -> w1
    stop <- w485 stop-if-true
    n169 = event shown="[0] Timeout" {
      selector: w481 -> [_ _ _ _ _ _ _ _ _ _ _]
      dyn-events: [_ _ _ _ _ _ _ _ _ _ _] -> w480
      timeout: 1000 -> [_ _ _ _ _ _ _ _ _ _ _]
      tunnel: w486 -> [w489 w497 w522 w571 w600 w607 w636 w641 w651 w657 w703]
      tunnel: [_ _ _ _ TRUE _ _ _ _ _ _] -> w485
      tunnel: [w489 w497 w519 w569 w596 w607 w633 w641 w649 w656 w704] -> w484
      tunnel: [w488 w493 w518 w568 w597 w603 w632 w638 w647 w654 _] -> w483
      tunnel: w482 -> [w488 w496 w517 w570 w598 w606 w631 w640 w648 w655 _]
      event Timeout {
        # "Timeout code can be added here for autosave or Lock Screen"
        n170 = event-data() -> ()  [unwired: 1 in, 1 out]
      }
      event "View": Shortcut Menu Activation? {
        n171 = event-data() -> ("CtlRef"=w503:refnum<vi>, "Coords"=w502:T18, "MenuRef"=w499:refnum<k9>)  [unwired: 1 in]
        n172 = invoke class="Tree (strict)" method="Point To Row Column"(reference=w503, error in=w496, "Point"=w502) -> (error out=w495:errorcluster, "Tag"=w501:string)  [unwired: 5 in, 6 out]
        n173 = call <vilib>:"IDtoNode.vi"("error in"=w495, "ID"=w501) -> ("error out"=w491:errorcluster, "invalid Id"=w498:bool, "node ref"=w500:T2)  [unwired: 7 in]
        n174 = case shown="False" w498 {
          tunnel: w500 -> [w508 _]
          tunnel: w499 -> [w507 _]
          tunnel: [w506 _] -> w494
          tunnel: [w505 _] -> w492
          tunnel: w491 -> [w504 w514]
          tunnel: [w504 w514] -> w490
          frame False {
            n175 = in-place {
              in-place-border: w507 -> [w511]
              in-place-border: [w509] -> w506
              n176 = in-place-dvr #7(w508) -> (w513:refnum<class "NISE_CEF_Node.lvclass">, w510:errorcluster)
              n177 = call-dynamic "ShortcutMenu.vi"("error in"=w510, "menu ref in"=w511, "node in"=w513) -> ("error out"=w509:errorcluster, "node out"=w512:refnum<class "NISE_CEF_Node.lvclass">)  [unwired: 6 in, 1 out]
              n178 = in-place-dvr #7(w512) -> (w505:errorcluster)  [unwired: 1 out]
            }
          }
          frame True {
          }
        }
        n179 = Merge Errors(w492, w494, w490) -> (w493:errorcluster)
        n180 = event-data() -> ()  [unwired: 2 in, 1 out]
      }
      event "View": Shortcut Menu Selection (User) {
        n181 = event-data() -> ("ItemPath"=w521:string, "CtlRef"=w524:refnum<vi>, "Coords"=w525:T18)  [unwired: 1 in]
        n182 = invoke class="Tree (strict)" method="Point To Row Column"(reference=w524, error in=w517, "Point"=w525) -> (error out=w516:errorcluster, "Tag"=w520:string)  [unwired: 5 in, 6 out]
        n183 = Match Pattern(string=w521, regular expression=":") -> (before substring=w523:string, after substring=w515:string)  [unwired: 1 in, 2 out]
        n184 = case shown="\"Add\"" w523 {
          selector: w523 -> [w527 _ _ _]
          tunnel: w515 -> [_ _ _ w552]
          tunnel: w522 -> [w534 w541 w547 w554]
          tunnel: w520 -> [w529 w539 w545 w553]
          tunnel: [w531 w538 w544 w550] -> w519
          tunnel: [w532 w537 w542 w548] -> w518
          tunnel: w516 -> [w533 w536 w543 w549]
          frame Default {
            n185 = Concatenate Strings(w527, ":" ("string"), w529) -> (w530:string)
            n186 = call <vilib>:"Send Local Message.vi"("message queue in"=w534, "message name"="CustomMenuAction" ("Message Name"), "message value"=w530, "error in"=w533) -> ("message queue out"=w531:T11, "error out"=w532:errorcluster)  [unwired: 9 in, 1 out]
          }
          frame "Remove" {
            n187 = call <vilib>:"Send Local Message.vi"("message queue in"=w541, "message name"="RemoveNode" ("Message Name"), "message value"=w539, "error in"=w536) -> ("message queue out"=w538:T11, "error out"=w537:errorcluster)  [unwired: 9 in, 1 out]
          }
          frame "Duplicate" {
            n188 = call <vilib>:"Send Local Message.vi"("message queue in"=w547, "message name"="Duplicate" ("Message Name"), "message value"=w545, "error in"=w543) -> ("message queue out"=w544:T11, "error out"=w542:errorcluster)  [unwired: 9 in, 1 out]
          }
          frame "Add" {
            n189 = Bundle By Name(cluster=T12 {"node type"="", "to add to"=""} ("input cluster"), "node type"=w552, "to add to"=w553) -> (w555:T12)
            n190 = Flatten To String(anything=w555) -> (data string=w556:string)  [unwired: 3 in, 2 out]
            n191 = call <vilib>:"Send Local Message.vi"("message queue in"=w554, "message name"="AddNode" ("Message Name"), "message value"=w556, "error in"=w549) -> ("message queue out"=w550:T11, "error out"=w548:errorcluster)  [unwired: 9 in, 1 out]
          }
        }
      }
      event "View": Drop {
        n192 = event-data() -> ("CtlRef"=w574:refnum<vi>, "Coords"=w573:T18)  [unwired: 1 in]
        n193 = invoke class="Tree (strict)" method="Point To Row Column"(reference=w574, error in=w570, "Point"=w573) -> (reference out=w572:refnum<vi>, error out=w567:errorcluster, "Tag"=w564:string)  [unwired: 5 in, 5 out]
        n194 = call <vilib>:"ValidDragDrop.vi"("error in"=w567, "Reorder"=TRUE, "drag over"=w564, "Tree Ref in"=w572) -> ("Error Out"=w559:errorcluster, "Accepted"=w562:bool, "Drag"=w566:string, "Tree Ref out"=w576:refnum<vi>, "Moved Node"=w560:T2, "Position"=w558:i32, "Parent Node"=w561:T2, "Parent"=w563:string)
        n195 = case shown="True" w562 {
          tunnel: w566 -> [_ w593]
          tunnel: w576 -> [_ w595]
          tunnel: [_ TRUE] -> w575
          tunnel: w563 -> [_ w591]
          tunnel: w571 -> [w578 w590]
          tunnel: [w578 w586] -> w569
          tunnel: [w577 w585] -> w568
          tunnel: w560 -> [_ w581]
          tunnel: w561 -> [_ w580]
          tunnel: w559 -> [w577 w582]
          tunnel: w558 -> [_ w579]
          frame False {
          }
          frame True {
            n196 = invoke class="Tree (strict)" method="Edit Tree Items.Move Item"(reference=w595, error in=w582, "tag"=w593, "New Parent"=w591) -> (error out=w583:errorcluster)  [unwired: 3 in, 6 out]
            n197 = Bundle By Name(cluster=T13 {"node ref"=refnum, "new parent"=refnum, "Index"=0} ("Cluster"), "Index"=w579, "node ref"=w581, "new parent"=w580) -> (w589:T13)
            n198 = Flatten To String(anything=w589, error in (no error)=w583) -> (data string=w588:string, error out=w584:errorcluster)  [unwired: 2 in, 1 out]
            n199 = call <vilib>:"Send Local Message.vi"("message queue in"=w590, "message name"="Move", "message value"=w588, "error in"=w584) -> ("message queue out"=w586:T11, "error out"=w585:errorcluster)  [unwired: 9 in, 1 out]
          }
        }
        n200 = event-data("Accepted?"=w575) -> ()  [unwired: 1 in, 1 out]
      }
      event "Exit": Value Change {
        # "Exit the application                                           >> Stop this message generator loop    Cleaning errors if the other loop stop this one"
        n201 = event-data() -> ()  [unwired: 1 in, 1 out]
        n202 = call <vilib>:"Send Local Message.vi"("message queue in"=w600, "message name"="Close", "error in"=w598) -> ("message queue out"=w596:T11, "error out"=w601:errorcluster)  [unwired: 10 in, 1 out]
        n203 = call <vilib>:"Clear Errors.vi"("error in (no error)"=w601) -> ("error out"=w597:errorcluster)  [unwired: 5 in, 1 out]
      }
      event "View": Drag Starting? {
        n204 = event-data() -> ("Data"=w613:T19, "CtlRef"=w615:refnum<vi>, "Coords"=w614:T18)  [unwired: 1 in]
        n205 = invoke class="Tree (strict)" method="Point To Row Column"(reference=w615, error in=w606, "Point"=w614) -> (error out=w605:errorcluster, "Tag"=w612:string)  [unwired: 5 in, 6 out]
        n206 = call <vilib>:"IDtoNode.vi"("error in"=w605, "ID"=w612) -> ("error out"=w604:errorcluster, "invalid Id"=w611:bool, "node ref"=w610:T2)  [unwired: 7 in]
        n207 = case shown="False" w611 {
          tunnel: w610 -> [w623 _]
          tunnel: [w620 TRUE ("Removable")] -> w608
          tunnel: w604 -> [w619 w629]
          tunnel: [w616 w629] -> w603
          frame False {
            n208 = in-place {
              in-place-border: [w626] -> w622
              in-place-border: w619 -> [w625]
              in-place-border: [w624] -> w618
              n209 = in-place-dvr #8(w623) -> (w628:refnum<class "NISE_CEF_Node.lvclass">)  [unwired: 1 out]
              n210 = call-dynamic "EditOptions.vi"("error in"=w625, "node in"=w628) -> ("error out"=w624:errorcluster, "edit options"=w626:T20, "node out"=w627:refnum<class "NISE_CEF_Node.lvclass">)  [unwired: 6 in, 1 out]
              n211 = in-place-dvr #8(w627) -> (w617:errorcluster)  [unwired: 1 out]
            }
            n212 = Unbundle By Name(w622) -> ("movable"=w621:bool)
            n213 = Merge Errors(w617, w618) -> (w616:errorcluster)
            n214 = Not(x=w621) -> (.not. x?=w620:bool)
          }
          frame True {
          }
        }
        n215 = event-data("Data"=w613, "Drag Mode"=enum32{"copy or move", "copy only", "move only"}."move only", "Discard?"=w608) -> ()  [unwired: 1 in, 1 out]
      }
      event "View": Value Change {
        n216 = event-data() -> ("NewVal"=w634:string)  [unwired: 1 in]
        n217 = call <vilib>:"Send Local Message.vi"("message queue in"=w636, "message name"="ActivateNode" ("Message Name"), "message value"=w634, "error in"=w631) -> ("message queue out"=w633:T11, "error out"=w632:errorcluster)  [unwired: 9 in, 1 out]
      }
      event "View": event type 3.0.xa000003a {
        n218 = event-data() -> ("CtlRef"=w646:refnum<vi>, "Coords"=w643:T18)  [unwired: 1 in]
        n219 = invoke class="Tree (strict)" method="Point To Row Column"(reference=w646, error in=w640, "Point"=w643) -> (reference out=w645:refnum<vi>, error out=w639:errorcluster, "Tag"=w644:string)  [unwired: 5 in, 5 out]
        n220 = call <vilib>:"ValidDragDrop.vi"("error in"=w639, "Reorder"=TRUE, "drag over"=w644, "Tree Ref in"=w645) -> ("Error Out"=w638:errorcluster, "Accepted"=w642:bool)  [unwired: 6 out]
        n221 = event-data("Accepted?"=w642) -> ()  [unwired: 1 in, 1 out]
      }
      event Panel Close? {
        # "Intercepts the upper right close panel operation to allow a smooth shutdown as opposed to immediately killing the app."
        n222 = event-data() -> ()  [unwired: 1 in, 1 out]
        n223 = call <vilib>:"Send Local Message.vi"("message queue in"=w651, "message name"="Close?", "error in"=w648) -> ("message queue out"=w649:T11, "error out"=w647:errorcluster)  [unwired: 10 in, 1 out]
        n224 = event-data("Discard?"=TRUE) -> ()  [unwired: 1 in, 1 out]
      }
      event Menu Selection (User) {
        # "#USERCFG It is needed to add a Case for Every item on the menu"
        n225 = event-data() -> ("ItemTag"=w653:string, "ItemPath"=w658:string)  [unwired: 1 in]
        n226 = case shown="\"_File:_New\"" w658 {
          selector: w658 -> [w662 _ _ _ _ _ _]
          tunnel: w657 -> [w667 w672 w677 w682 w687 w692 w701]
          tunnel: [w667 w668 w673 w678 w683 w688 w698] -> w656
          tunnel: w655 -> [w664 w670 w675 w680 w685 w690 w697]
          tunnel: [w663 w669 w674 w679 w684 w689 w695] -> w654
          tunnel: w653 -> [w661 _ _ _ _ _ _]
          frame Default {
            n227 = Concatenate Strings(w661, "::" ("string"), w662) -> (w660:string)
            n228 = call <vilib>:"NISE_error generator.vi"("error in"=w664, "source"="configuration tool main.vi", "append error message"=w660, "error code (0)"=538506) -> ("error out"=w663:errorcluster)  [unwired: 5 in]
          }
          frame "_File:_New" {
            n229 = call <vilib>:"Send Local Message.vi"("message queue in"=w672, "message name"="New?" ("Message Name"), "error in"=w670) -> ("message queue out"=w668:T11, "error out"=w669:errorcluster)  [unwired: 10 in, 1 out]
          }
          frame "_File:_Open" {
            n230 = call <vilib>:"Send Local Message.vi"("message queue in"=w677, "message name"="Open?" ("Message Name"), "error in"=w675) -> ("message queue out"=w673:T11, "error out"=w674:errorcluster)  [unwired: 10 in, 1 out]
          }
          frame "_File:_Save" {
            n231 = call <vilib>:"Send Local Message.vi"("message queue in"=w682, "message name"="Save" ("Message Name"), "error in"=w680) -> ("message queue out"=w678:T11, "error out"=w679:errorcluster)  [unwired: 10 in, 1 out]
          }
          frame "_File:Save As..." {
            n232 = call <vilib>:"Send Local Message.vi"("message queue in"=w687, "message name"="SaveAs" ("Message Name"), "error in"=w685) -> ("message queue out"=w683:T11, "error out"=w684:errorcluster)  [unwired: 10 in, 1 out]
          }
          frame "_File:_Exit" {
            n233 = call <vilib>:"Send Local Message.vi"("message queue in"=w692, "message name"="Close?" ("Message Name"), "error in"=w690) -> ("message queue out"=w688:T11, "error out"=w689:errorcluster)  [unwired: 10 in, 1 out]
          }
          frame "_Tools:Multiple Parameter Editor" {
            n234 = call <vilib>:"Send Local Message.vi"("message queue in"=w701, "message name"="CleansubPanel", "error in"=w697) -> ("message queue out"=w700:T11, "error out"=w696:errorcluster)  [unwired: 10 in, 1 out]
            n235 = call <vilib>:"Send Local Message.vi"("message queue in"=w700, "message name"="Custom View" ("Message Name"), "message value"="Multiple Variable Editor" ("Message Name"), "error in"=w696) -> ("message queue out"=w698:T11, "error out"=w695:errorcluster)  [unwired: 9 in, 1 out]
          }
        }
      }
      event User Event {
        n236 = event-data() -> ("node ref"=w702:T2)  [unwired: 1 in]
        n237 = call <vilib>:"NodetoID.vi"("node ref"=w702) -> ("ID"=w705:string)  [unwired: 9 in, 1 out]
        n238 = call <vilib>:"Send Local Message.vi"("message queue in"=w703, "message name"="NodeDataChange", "message value"=w705) -> ("message queue out"=w704:T11)  [unwired: 10 in, 2 out]
      }
    }
    n239 = call "Error.vi"("error in (no error)"=w483, "message queue in"=w484) -> ()  [unwired: 9 in, 1 out]
  }
  n240 = Unregister For Events(event registration refnum=w1) -> (error out=w2:errorcluster)  [unwired: 1 in]
  n241 = Merge Errors(w2, w7) -> (w3:errorcluster)
  n242 = call <vilib>:"DestroyStandardEvents.vi"("error in"=w3, "standard events"=w6) -> ()  [unwired: 9 in, 1 out]
